vi "State_Machine.vi"(8 "error in (no error)":errorcluster caption="entrée d'erreur (pas d'erreur)", 11 "Delay en entrée":refnum<class "P2056_Get_IMEI.lvclass">) -> (0 "error out":errorcluster caption="sortie d'erreur", 2 "Json_String":string, 3 "Delay en sortie":refnum<class "P2056_Get_IMEI.lvclass">)   [LabVIEW 2020, in "Library Test.lvlib" / "P2056_Get_IMEI.lvclass"]
uses:
  P2056_Get_IMEI.lvclass
  C:/Users/ngarcin/OneDrive - Altyor/Standard TB/Suite TB45/Class/Test/Test (Default)/Test (Default).lvclass
  Commun VI/TypeDef/Variable Printable.ctl
  Read CSV File/CSV_File (Default)/Class CSV_File.lvclass
  C:/Users/ngarcin/OneDrive - Altyor/Standard TB/Suite TB45/Class/Read CSV File/Class File (Default)/Class File (Default).lvclass
  JSON API/JSON Value/Set from JSON string.vi
  JSON API/JSON Value/JSON Value.lvclass
  JSON API/Variant JSON/Variant JSON.lvlib
  JSON API/Get Polymorphic/JSON GetSet.lvlib
  Commun VI/Library Commun.lvlib
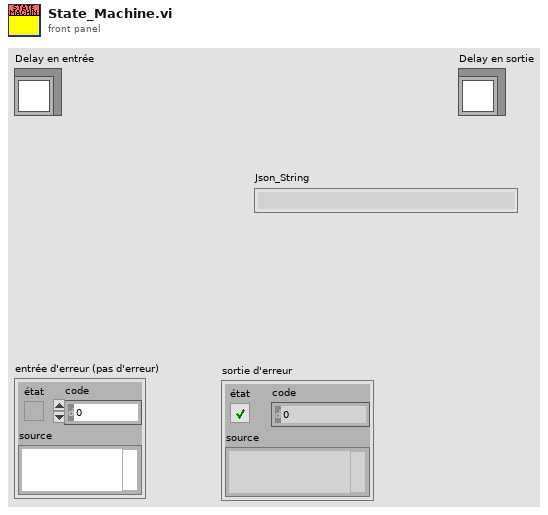
[diagram p1: front panel]
types:
  T1 = typedef "Variable Printable.ctl" = string
  T2 = enum16{"Get Variable", "Get All Variables", "Set Variable", "Delete Variable", "Delete All Variable"}
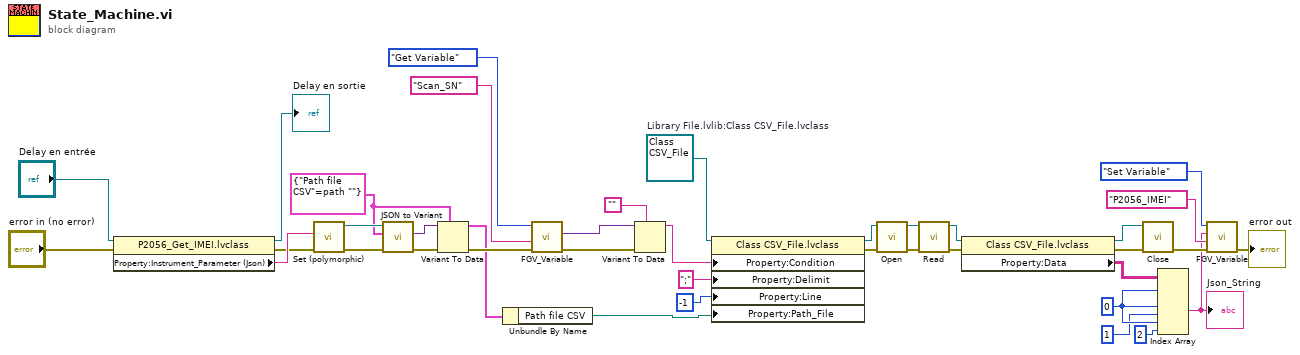
[diagram p0: block diagram]
diagram:
  w3 = refnum<class "Class CSV_File.lvclass"> refnum  # Library File.lvlib:Class CSV_File.lvclass
  w13 = 0 ("indice (ligne)")
  w31 = cluster{"Path file CSV":path} {"Path file CSV"=path ""}
  n1 = property class="P2056_Get_IMEI.lvclass"(reference="Delay en entrée", error in="error in (no error)") -> (reference out=→"Delay en sortie":refnum<class "P2056_Get_IMEI.lvclass">, error out=w32:errorcluster, "Property:Instrument_Parameter (Json)"=w34:string)
  n2 = call-poly "Set (polymorphic).vi"("error in (no error)"=w32, "JSON stream"=w34) -> ("error out"=w36:errorcluster, "JSON Value out"=w38:refnum<class "JSON Value.lvclass">)  [unwired: 7 in, 1 out]
  n3 = call "JSON to Variant.vi"("error in (no error)"=w36, "Variant (Data Type)"=w31, "JSON Value"=w38) -> ("error out"=w37:errorcluster, "Variant out"=w35:variant)  [unwired: 7 in]
  n4 = Variant To Data(error in=w37, type=w31, Variant=w35) -> (data=w18:cluster{"Path file CSV":path}, error out=w26:errorcluster)
  n5 = Unbundle By Name(w18) -> ("Path file CSV"=w2:path)
  n6 = call "FGV_Variable.vi"("error in (no error)"=w26, "Variable"=T1 "Scan_SN", "Function"=T2."Get Variable") -> ("error out"=w25:errorcluster, "Data Out"=w19:variant)  [unwired: 6 in, 1 out]
  n7 = Variant To Data(error in=w25, type="", Variant=w19) -> (data=w1:string)  [unwired: 1 out]
  n8 = property class="Class CSV_File.lvclass"(reference=w3, "Property:Condition"=w1, "Property:Delimit"=";" ("Delimit"), "Property:Line"=i16 -1 ("Line"), "Property:Path_File"=w2) -> (reference out=w15:refnum<class "Class CSV_File.lvclass">, error out=w14:errorcluster)  [unwired: 1 in]
  n9 = call-dynamic "Open.vi"("error in (no error)"=w14, "Class CSV_File (Default) en entrée"=w15) -> ("error out"=w17:errorcluster, "Class CSV_File (Default) en sortie"=w16:refnum<class "Class CSV_File.lvclass">)  [unwired: 8 in]
  n10 = call-dynamic "Read.vi"("error in (no error)"=w17, "Class CSV_File (Default) en entrée"=w16) -> ("error out"=w23:errorcluster, "Class CSV_File (Default) en sortie"=w21:refnum<class "Class CSV_File.lvclass">)  [unwired: 8 in]
  n11 = property class="Class CSV_File.lvclass"(reference=w21, error in=w23) -> (reference out=w20:refnum<class "Class CSV_File.lvclass">, error out=w22:errorcluster, "Property:Data"=w10:string[][])
  n12 = call-dynamic "Close.vi"("error in (no error)"=w22, "Class CSV_File (Default) en entrée"=w20) -> ("error out"=w6:errorcluster)  [unwired: 8 in, 1 out]
  n13 = Index Array(array=w10, index (row) #1=w13, index (row) #2=w13, index (col) #2=1 ("indice désactivé (col)"), index (row) #3=w13, index (col) #3=2 ("indice désactivé (col)")) -> (element #2=w4:string)  [unwired: 1 in, 2 out]
  "Json_String" <- w4
  n14 = call "FGV_Variable.vi"("error in (no error)"=w6, "Variable"=T1 "P2056_IMEI", "Data In"=w4, "Function"=T2."Set Variable") -> ("error out"=→"error out":errorcluster)  [unwired: 5 in, 2 out]
